vi "Finish.vi"   [LabVIEW 2014]
doc: "This VI is called just before exiting. It is expected to close I/O refnum, save collected data, etc."
uses:
  <vilib>/Rock Robotics/WPI/Joystick/WPI_JoystickGetSetRefNum.vi
types:
  T1 = typedef "WPI_JoystickDevRef.ctl" = cluster{"Device":T2}
  T2 = typedef "WPI_JoystickDeviceEnum.ctl" = enum16{"USB 0", "USB 1", "USB 2", "USB 3", "USB 4", "USB 5"}
  T3 = typedef "WPI_EncoderDevRef.ctl" = cluster{"DevStatus":errorcluster, "EncoderIndex":T4, "CounterIndex":T5, "DistancePerCount":dbl, "Decoding Type":T6}
  T4 = typedef "FPGA_EncoderIdx.ctl" = enum8{"Enc 0", "Enc 1", "Enc 2", "Enc 3", "Enc 4", "Enc 5", "Enc 6", "Enc 7", "Invalid"}
  T5 = typedef "FPGA_CounterCtrSystemIndex.ctl" = enum8{"Ctr 0", "Ctr 1", "Ctr 2", "Ctr 3", "Ctr 4", "Ctr 5", "Ctr 6", "Ctr 7", "Invalid"}
  T6 = typedef "WPI_EncoderType.ctl" = enum16{"1x", "2x", "4x"}
  T7 = typedef "WPI_MotorControlDeviceRef.ctl" = cluster{"DeviceStatus":errorcluster, "Type":T8, "PWM":cluster{"Controller":T9, "PWM Channel":T10, "DeadBand":T11}, "CAN":cluster{"Device Number":u8, "Control Mode":T12, "Semaphore":T13, "Max Vout":dbl, "TalonSRX Control Mode":T14}, "Invert":bool, "TransformRef":T15, "InvTransformRef":T15}
  T8 = typedef "WPI_MotorControlType.ctl" = enum16{"PWM", "CAN", "CANTalonSRX"}
  T9 = typedef "FPGA_TypedefDigitalModule.ctl" = enum16{"Controller 1"}
  T10 = typedef "FPGA_DIOPWMChannel.ctl" = enum8{"PWM 0", "PWM 1", "PWM 2", "PWM 3", "PWM 4", "PWM 5", "PWM 6", "PWM 7", "PWM 8", "PWM 9", "PWM MXP 0", "PWM MXP 1", "PWM MXP 2", "PWM MXP 3", "PWM MXP 4", "PWM MXP 5", "PWM MXP 6", "PWM MXP 7", "PWM MXP 8", "PWM MXP 9", "Invalid"}
  T11 = typedef "WPI_PWMDeadband.ctl" = cluster{"Name":string, "maxPositivePwm":i32, "minPositivePwm":i32, "centerPwm":i32, "maxNegativePwm":i32, "minNegativePwm":i32, "angularRange":u16}
  T12 = typedef "WPI_CANJaguar_ControlMode.ctl" = enum8{"Percent VBus", "Current", "Speed", "Position", "Voltage"}
  T13 = typedef "Semaphore RefNum" = refnum<k1>
  T14 = typedef "WPI_CANTalonSRX_APIControlMode.ctl" = enum8{"Percent VBus", "Speed", "Position", "Slave", "Unchanged / Invalid"}
  T15 = typedef "WPI_PWMTransform_ConPane.ctl" = refnum<vi>
  T16 = typedef "WPI_GyroDevRef.ctl" = cluster{"DevStatus":errorcluster, "Analog Module":T17, "Analog Channel":T18, "Offset":dbl, "Gain (VoltsPerDegree/Second)":dbl}
  T17 = typedef "FPGA_TypedefAnalogModule.ctl" = enum16{"Controller 1"}
  T18 = typedef "FPGA_AIChannel.ctl" = enum8{"AI 0", "AI 1", "AI 2", "AI 3", "AI MXP 0", "AI MXP 1", "AI MXP 2", "AI MXP 3", "Invalid"}
  T19 = typedef "WPI_SolenoidDevRef.ctl" = cluster{"DevStatus":errorcluster, "Pneumatics Control Module":u8, "Forward Solenoid Channel":T20, "Reverse Solenoid Channel":T20}
  T20 = typedef "WPI_SolenoidChannel.ctl" = enum8{"Solenoid 0", "Solenoid 1", "Solenoid 2", "Solenoid 3", "Solenoid 4", "Solenoid 5", "Solenoid 6", "Solenoid 7", "Invalid"}
  T21 = typedef "WPI_RelayDevRef.ctl" = cluster{"DevStatus":errorcluster, "Relay Channel":T22, "Controller":T9, "Relay Direction":T23}
  T22 = typedef "FPGA_DIORelayChannel.ctl" = enum8{"Relay 0", "Relay 1", "Relay 2", "Relay 3", "Invalid"}
  T23 = typedef "WPI_RelayDirection.ctl" = enum16{"Both directions", "Forward only", "Reverse only"}
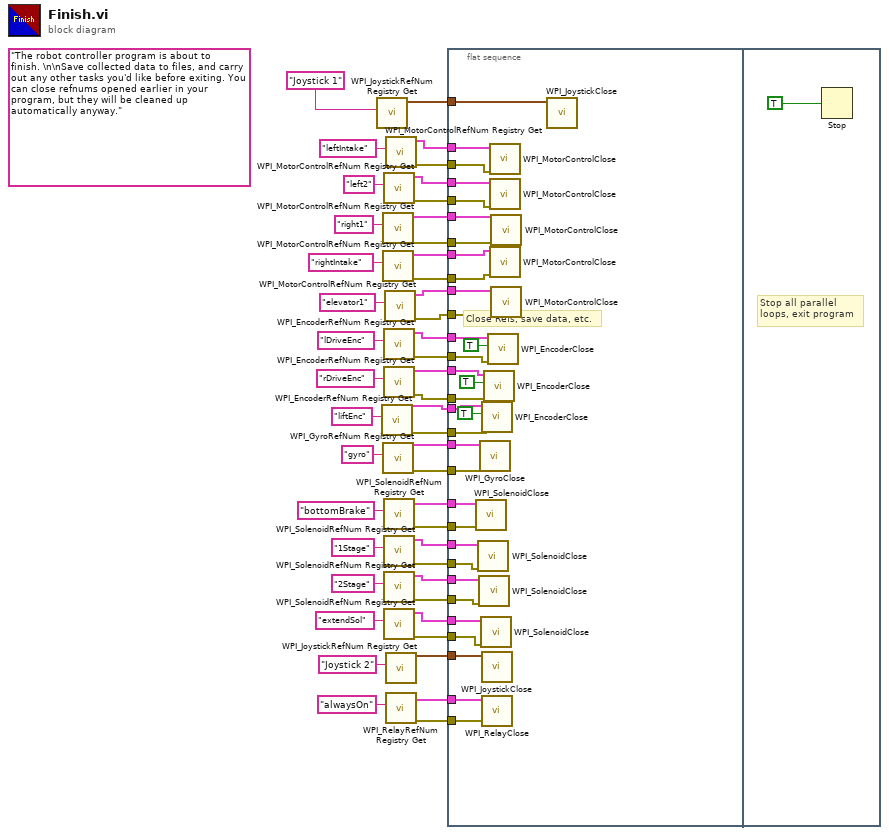
[diagram p0: block diagram]
diagram:
  (unwired) "The robot controller program is about to finish. \n\nSave collected data to files, and carry out any other tasks you'd like before exiting. You can close refnums opened earlier in your program, but they will be cleaned up automatically anyway."
  n1 = call <vilib>:"WPI_JoystickRefNum Registry Get.vi"("refnum name"="Joystick 1") -> ("JoystickDevRef"=w45:T1)  [unwired: 1 in, 9 out]
  n2 = call <vilib>:"WPI_EncoderRefNum Registry Get.vi"("refnum name"="liftEnc") -> ("error out"=w31:errorcluster, "EncoderDevRef"=w32:T3)  [unwired: 9 in]
  n3 = call <vilib>:"WPI_MotorControlRefNum Registry Get.vi"("refnum name"="right1") -> ("error out"=w23:errorcluster, "MotorControlDevRef"=w24:T7)  [unwired: 9 in]
  n4 = call <vilib>:"WPI_MotorControlRefNum Registry Get.vi"("refnum name"="rightIntake") -> ("error out"=w21:errorcluster, "MotorControlDevRef"=w22:T7)  [unwired: 9 in]
  n5 = call <vilib>:"WPI_GyroRefNum Registry Get.vi"("refnum name"="gyro") -> ("error out"=w29:errorcluster, "GyroDevRef"=w30:T16)  [unwired: 9 in]
  n6 = call <vilib>:"WPI_MotorControlRefNum Registry Get.vi"("refnum name"="left2") -> ("error out"=w25:errorcluster, "MotorControlDevRef"=w26:T7)  [unwired: 9 in]
  n7 = call <vilib>:"WPI_EncoderRefNum Registry Get.vi"("refnum name"="lDriveEnc") -> ("error out"=w35:errorcluster, "EncoderDevRef"=w36:T3)  [unwired: 9 in]
  n8 = call <vilib>:"WPI_EncoderRefNum Registry Get.vi"("refnum name"="rDriveEnc") -> ("error out"=w33:errorcluster, "EncoderDevRef"=w34:T3)  [unwired: 9 in]
  n9 = call <vilib>:"WPI_SolenoidRefNum Registry Get.vi"("refnum name"="bottomBrake") -> ("error out"=w16:errorcluster, "SolenoidDevRef"=w17:T19)  [unwired: 9 in]
  n10 = call <vilib>:"WPI_SolenoidRefNum Registry Get.vi"("refnum name"="1Stage") -> ("error out"=w14:errorcluster, "SolenoidDevRef"=w15:T19)  [unwired: 9 in]
  n11 = call <vilib>:"WPI_SolenoidRefNum Registry Get.vi"("refnum name"="2Stage") -> ("error out"=w12:errorcluster, "SolenoidDevRef"=w13:T19)  [unwired: 9 in]
  n12 = call <vilib>:"WPI_SolenoidRefNum Registry Get.vi"("refnum name"="extendSol") -> ("error out"=w10:errorcluster, "SolenoidDevRef"=w11:T19)  [unwired: 9 in]
  n13 = call <vilib>:"WPI_MotorControlRefNum Registry Get.vi"("refnum name"="elevator1") -> ("error out"=w19:errorcluster, "MotorControlDevRef"=w20:T7)  [unwired: 9 in]
  n14 = call <vilib>:"WPI_MotorControlRefNum Registry Get.vi"("refnum name"="leftIntake") -> ("error out"=w27:errorcluster, "MotorControlDevRef"=w28:T7)  [unwired: 9 in]
  n15 = call <vilib>:"WPI_JoystickRefNum Registry Get.vi"("refnum name"="Joystick 2") -> ("JoystickDevRef"=w5:T1)  [unwired: 1 in, 9 out]
  n16 = call <vilib>:"WPI_RelayRefNum Registry Get.vi"("refnum name"="alwaysOn") -> ("error out"=w2:errorcluster, "RelayDevRef"=w3:T21)  [unwired: 9 in]
  n17 = flat-sequence {
    tunnel: w45 -> [w79]
    tunnel: w36 -> [w78]
    tunnel: w35 -> [w77]
    tunnel: w34 -> [w75]
    tunnel: w33 -> [w74]
    tunnel: w32 -> [w73]
    tunnel: w31 -> [w72]
    tunnel: w30 -> [w71]
    tunnel: w29 -> [w70]
    tunnel: w28 -> [w69]
    tunnel: w27 -> [w68]
    tunnel: w26 -> [w67]
    tunnel: w25 -> [w66]
    tunnel: w24 -> [w65]
    tunnel: w23 -> [w64]
    tunnel: w22 -> [w63]
    tunnel: w21 -> [w62]
    tunnel: w20 -> [w61]
    tunnel: w19 -> [w60]
    tunnel: w17 -> [w57]
    tunnel: w16 -> [w56]
    tunnel: w15 -> [w55]
    tunnel: w14 -> [w54]
    tunnel: w13 -> [w53]
    tunnel: w12 -> [w52]
    tunnel: w11 -> [w51]
    tunnel: w10 -> [w50]
    tunnel: w5 -> [w49]
    tunnel: w3 -> [w48]
    tunnel: w2 -> [w47]
    frame #0 {
      # "Close Refs, save data, etc."
      n18 = call <vilib>:"WPI_SolenoidClose.vi"("error in (no error)"=w56, "SolenoidDevRef"=w57) -> ()  [unwired: 9 in, 1 out]
      n19 = call <vilib>:"WPI_SolenoidClose.vi"("error in (no error)"=w54, "SolenoidDevRef"=w55) -> ()  [unwired: 9 in, 1 out]
      n20 = call <vilib>:"WPI_SolenoidClose.vi"("error in (no error)"=w52, "SolenoidDevRef"=w53) -> ()  [unwired: 9 in, 1 out]
      n21 = call <vilib>:"WPI_GyroClose.vi"("error in (no error)"=w70, "GyroDevRef"=w71) -> ()  [unwired: 9 in, 1 out]
      n22 = call <vilib>:"WPI_SolenoidClose.vi"("error in (no error)"=w50, "SolenoidDevRef"=w51) -> ()  [unwired: 9 in, 1 out]
      n23 = call <vilib>:"WPI_EncoderClose.vi"("error in (no error)"=w72, "Close Dependencies"=TRUE, "EncoderDevRef"=w73) -> ()  [unwired: 8 in, 1 out]
      n24 = call <vilib>:"WPI_JoystickClose.vi"("JoystickDevRef"=w49) -> ()  [unwired: 11 out]
      n25 = call <vilib>:"WPI_RelayClose.vi"("error in (no error)"=w47, "RelayDevRef"=w48) -> ()  [unwired: 9 in, 1 out]
      n26 = call <vilib>:"WPI_EncoderClose.vi"("error in (no error)"=w74, "Close Dependencies"=TRUE, "EncoderDevRef"=w75) -> ()  [unwired: 8 in, 1 out]
      n27 = call <vilib>:"WPI_EncoderClose.vi"("error in (no error)"=w77, "Close Dependencies"=TRUE, "EncoderDevRef"=w78) -> ()  [unwired: 8 in, 1 out]
      n28 = call <vilib>:"WPI_MotorControlClose.vi"("error in (no error)"=w68, "MotorControlDevRef"=w69) -> ()  [unwired: 9 in, 1 out]
      n29 = call <vilib>:"WPI_MotorControlClose.vi"("error in (no error)"=w66, "MotorControlDevRef"=w67) -> ()  [unwired: 9 in, 1 out]
      n30 = call <vilib>:"WPI_MotorControlClose.vi"("error in (no error)"=w62, "MotorControlDevRef"=w63) -> ()  [unwired: 9 in, 1 out]
      n31 = call <vilib>:"WPI_MotorControlClose.vi"("error in (no error)"=w64, "MotorControlDevRef"=w65) -> ()  [unwired: 9 in, 1 out]
      n32 = call <vilib>:"WPI_MotorControlClose.vi"("error in (no error)"=w60, "MotorControlDevRef"=w61) -> ()  [unwired: 9 in, 1 out]
      n33 = call <vilib>:"WPI_JoystickClose.vi"("JoystickDevRef"=w79) -> ()  [unwired: 11 out]
    }
    frame #1 {
      # "Stop all parallel\nloops, exit program"
      n34 = Stop(stop? (T)=TRUE ("Quit")) -> ()
    }
  }
